vi "Fill Meter.vi"(9 "Pour Size":string, 11 "Fill Meter Reference":refnum<vi>) -> ()   [LabVIEW 2020]
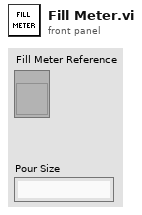
[diagram p1: front panel]
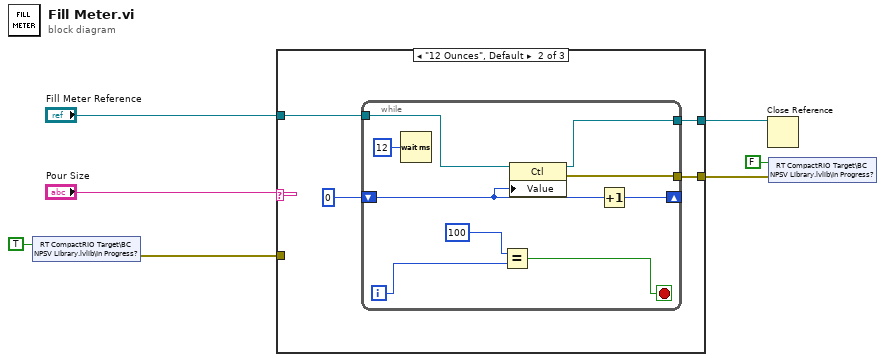
[diagram p0: block diagram]
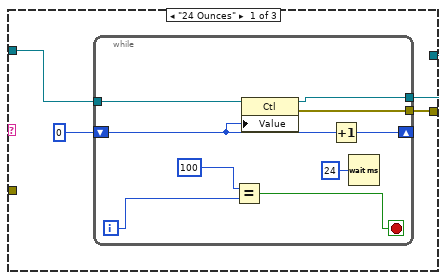
[diagram p2: hidden frame]
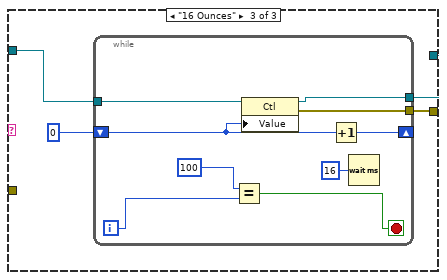
[diagram p3: hidden frame]
diagram:
  n1 = shared-variable "RT CompactRIO Target\\BC NPSV Library.lvlib\\In Progress?"(TRUE ("In Progress?")) -> (error out=w1:errorcluster)  [unwired: 1 in]
  n2 = case shown="\"12 Ounces\", Default" "Pour Size" {
    tunnel: "Fill Meter Reference" -> [w11 w24 w37]
    tunnel: [w9 w22 w35] -> w5
    tunnel: [w8 w21 w34] -> w3
    tunnel: w1 -> [_ _ _]
    frame "24 Ounces" {
      n3 = while {
        tunnel: w11 -> [w20]
        shift-right: [w16] -> _
        shift-left: 0 -> [w17]
        tunnel: [w13] -> w9
        tunnel: [w12] -> w8
        i -> [w19]
        stop <- w15 stop-if-true
        n4 = Equal?(x=100, y=w19) -> (x = y?=w15:bool)
        n5 = property class="Ctl"(reference=w20, "Value"=w17) -> (reference out=w13:refnum<vi>, error out=w12:errorcluster)  [unwired: 1 in]
        n6 = Increment(x=w17) -> (x+1=w16:i32)
        n7 = Wait (ms)(milliseconds to wait=u32 24) -> ()  [unwired: 1 out]
      }
    }
    frame "12 Ounces", Default {
      n8 = while {
        tunnel: w24 -> [w33]
        shift-right: [w29] -> _
        shift-left: 0 -> [w30]
        tunnel: [w26] -> w22
        tunnel: [w25] -> w21
        i -> [w32]
        stop <- w28 stop-if-true
        n9 = Wait (ms)(milliseconds to wait=u32 12) -> ()  [unwired: 1 out]
        n10 = Equal?(x=100, y=w32) -> (x = y?=w28:bool)
        n11 = property class="Ctl"(reference=w33, "Value"=w30) -> (reference out=w26:refnum<vi>, error out=w25:errorcluster)  [unwired: 1 in]
        n12 = Increment(x=w30) -> (x+1=w29:i32)
      }
    }
    frame "16 Ounces" {
      n13 = while {
        tunnel: w37 -> [w46]
        shift-right: [w42] -> _
        shift-left: 0 -> [w43]
        tunnel: [w39] -> w35
        tunnel: [w38] -> w34
        i -> [w45]
        stop <- w41 stop-if-true
        n14 = Equal?(x=100, y=w45) -> (x = y?=w41:bool)
        n15 = property class="Ctl"(reference=w46, "Value"=w43) -> (reference out=w39:refnum<vi>, error out=w38:errorcluster)  [unwired: 1 in]
        n16 = Increment(x=w43) -> (x+1=w42:i32)
        n17 = Wait (ms)(milliseconds to wait=u32 16) -> ()  [unwired: 1 out]
      }
    }
  }
  n18 = Close Reference(reference=w5) -> ()  [unwired: 1 in, 1 out]
  n19 = shared-variable "RT CompactRIO Target\\BC NPSV Library.lvlib\\In Progress?"(FALSE ("In Progress?"), error in=w3) -> ()  [unwired: 1 out]
